vi "Factory (JSON).vi"(8 "error in (no error)":errorcluster, 10 "JSON":string) -> (0 "error out":errorcluster, 3 "BLRL Source":refnum<class "BluelinesRedlines Source.lvclass">)   [LabVIEW 2020, in "VolatusGUI.lvlib" / "BluelinesRedlines Source.lvclass"]
uses:
  BluelinesRedlines Source.lvclass
  <vilib>/JDP Science/JSONtext/Next JSON Value.vi
  <vilib>/JDP Science/JSONtext/String Subset.vi
  <vilib>/JDP Science/JSONtext/Parsing/Advance past next JSON Value (inlined COPY).vi
  <vilib>/JDP Science/JSONtext/Parsing/Advance past whitespace.vi
  <vilib>/JDP Science/JSONtext/Parsing/Advance past String.vi
  <vilib>/JDP Science/JSONtext/Parsing/Advance past Number.vi
  <vilib>/JDP Science/JSONtext/Parsing/Advance past Line Ending.vi
  <vilib>/JDP Science/JSONtext/Parsing/Parse Full Path or Item Name.vi
  <vilib>/JDP Science/JSONtext/Parsing/Advance past Array.vi
  <vilib>/JDP Science/JSONtext/Parsing/Advance past Object.vi
  <vilib>/JDP Science/JSONtext/support/Error Cluster From Code.vi
  <vilib>/JDP Science/JSONtext/Offset/Find Item Locations by Path.vi
  <vilib>/JDP Science/JSONtext/JSONtext.lvlib
  7d19b383-de84-4a10-87c0-2ed965dc0f24.vi
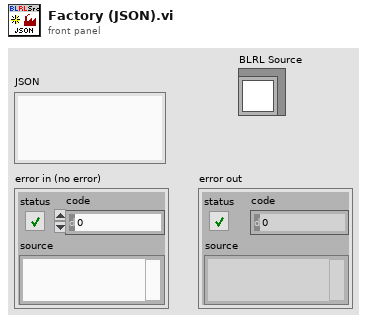
[diagram p1: front panel]
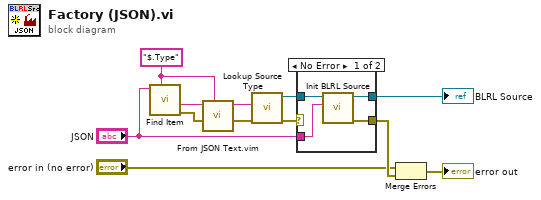
[diagram p0: block diagram]
diagram:
  w2 = "$.Type" ("$Path or Item Name")
  n1 = call <vilib>:"Find Item.vi"("$Path or Item Name"=w2, "JSON"="JSON") -> ("error out"=w10:errorcluster, "<JSON>"=w3:string)  [unwired: 6 in, 2 out]
  n2 = call "From JSON Text.vim"("Data Type and Default Value"=w2, "error in (no error)"=w10, "JSON"=w3) -> ("error out"=w4:errorcluster, "Data out"=w1:string)  [unwired: 7 in]
  n3 = call "Lookup Source Type.vi"("error in (no error)"=w4, "Source Type"=w1) -> ("error out"=w12:errorcluster, "Source"=w11:refnum<class "BluelinesRedlines Source.lvclass">)  [unwired: 8 in]
  n4 = case shown="No Error" w12 {
    selector: w12 -> [_ w17]
    tunnel: w11 -> [w16 _]
    tunnel: "JSON" -> [w15 _]
    tunnel: [w14 _] -> w8
    tunnel: [w13 w17] -> w7
    frame No Error {
      n5 = call-dynamic "Init BLRL Source.vi"("Config JSON"=w15, "BluelinesRedlines Source in"=w16) -> ("error out"=w13:errorcluster, "BluelinesRedlines Source out"=w14:refnum<class "BluelinesRedlines Source.lvclass">)  [unwired: 8 in]
    }
    frame Error {
    }
  }
  "BLRL Source" <- w8
  n6 = Merge Errors("error in (no error)", w7) -> (→"error out":errorcluster)
